vi "acc_to_distance.vi"(0 "Acc_x":dbl, 5 "Acc_y":dbl, 7 "Acc_z":dbl, 9 "distance_in":dbl[](array[numeric]), 11 "velocity_in":dbl[](array[numeric])) -> (4 "distance_out":dbl[](array[numeric]), 6 "velocity_out":dbl[](array[numeric]))   [LabVIEW 2015]
panel:
  out "position_z_out":dbl
  out "position_y_out":dbl
  out "position_x_out":dbl
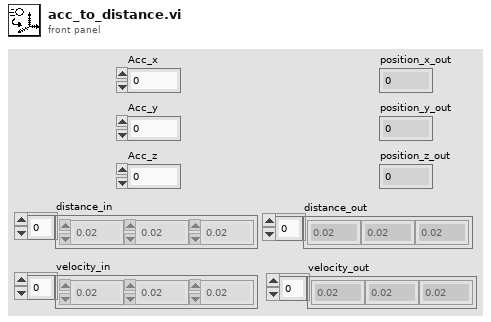
[diagram p1: front panel]
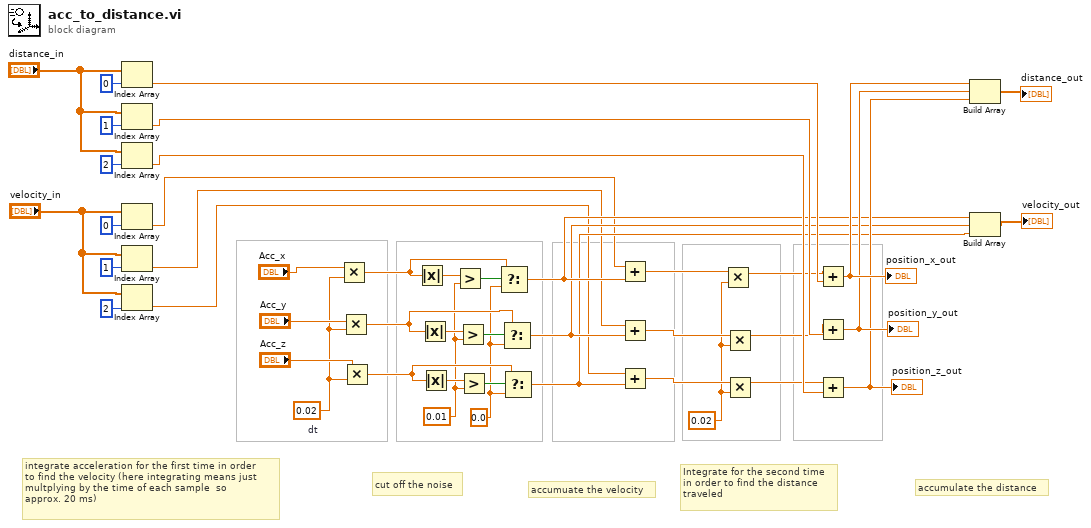
[diagram p0: block diagram]
diagram:
  w4 = 0.02 ("y")
  w13 = 0.0 ("f")
  w14 = 0.01 ("y")
  w41 = 0.02  # dt
  # "accumulate the distance"
  # "accumuate the velocity"
  # "cut off the noise"
  # "Integrate for the second time\nin order to find the distance\ntraveled"
  # "integrate acceleration for the first time in order\nto find the velocity (here integrating means just \nmultplying by the time of each sample  so \napprox. 20 ms)"
  n1 = Index Array(array="distance_in", index=0) -> (element=w31:dbl)
  n2 = Index Array(array="distance_in", index=1) -> (element=w30:dbl)
  n3 = Index Array(array="distance_in", index=2) -> (element=w29:dbl)
  n4 = Index Array(array="velocity_in", index=0) -> (element=w1:dbl)
  n5 = Index Array(array="velocity_in", index=1) -> (element=w2:dbl)
  n6 = Index Array(array="velocity_in", index=2) -> (element=w3:dbl)
  n7 = Multiply(x="Acc_x", y=w41) -> (x*y=w40:dbl)
  n8 = Multiply(x="Acc_y", y=w41) -> (x*y=w39:dbl)
  n9 = Multiply(x="Acc_z", y=w41) -> (x*y=w38:dbl)
  n10 = Absolute Value(x=w40) -> (abs(x)=w15:dbl)
  n11 = Absolute Value(x=w39) -> (abs(x)=w16:dbl)
  n12 = Absolute Value(x=w38) -> (abs(x)=w18:dbl)
  n13 = Greater?(x=w15, y=w14) -> (0:w20:bool)
  n14 = Greater?(x=w16, y=w14) -> (0:w19:bool)
  n15 = Greater?(x=w18, y=w14) -> (0:w17:bool)
  n16 = Select(t=w40, s=w20, f=w13) -> (s? t:f=w12:dbl)
  n17 = Select(t=w39, s=w19, f=w13) -> (s? t:f=w11:dbl)
  n18 = Select(t=w38, s=w17, f=w13) -> (s? t:f=w10:dbl)
  n19 = Add(x=w1, y=w12) -> (x+y=w37:dbl)
  n20 = Add(x=w2, y=w11) -> (x+y=w8:dbl)
  n21 = Add(x=w3, y=w10) -> (x+y=w36:dbl)
  n22 = Multiply(x=w37, y=w4) -> (x*y=w7:dbl)
  n23 = Multiply(x=w8, y=w4) -> (x*y=w6:dbl)
  n24 = Multiply(x=w36, y=w4) -> (x*y=w5:dbl)
  n25 = Add(x=w7, y=w31) -> (x+y=w24:dbl)
  "position_x_out" <- w24
  n26 = Add(x=w6, y=w30) -> (x+y=w23:dbl)
  "position_y_out" <- w23
  n27 = Add(x=w5, y=w29) -> (x+y=w22:dbl)
  "position_z_out" <- w22
  n28 = Build Array(w24, w23, w22) -> (→"distance_out":dbl[])
  n29 = Build Array(w12, w11, w10) -> (→"velocity_out":dbl[])
